vi "Combine Log of Mantissa and Exponent (SGL).vi"(5 "Exponent of 2":u8, 7 "10Log (Mantissa)":fxp<+/-,18,8>, 9 "Input Valid":bool=TRUE) -> (6 "Logarithm":fxp<+/-,34,12> format="%.26g", 10 "Output Valid":bool)   [LabVIEW 2012]
doc: "This VI implements the arithmetic of 10* log(M) + 10*log2* N\n\nOutput= 10Log(Matissa) + 3.01 *N\n\n<b> Resources Used: DSP48E</b>\n<b> Latency = 5 Ticks </b>"
uses:
  <vilib>/rvi/FXPMathLib/basic elements/DSP48E/simVIs/niFpgaDsp48eSimulationState.ctl
  <vilib>/rvi/FXPMathLib/basic elements/DSP48E/subVIs/niFpgaDsp48eType.ctl
  <vilib>/rvi/FXPMathLib/basic elements/DSP48E/subVIs/niFpgaDsp48eAlumodeOpmodeCarryinselState.ctl
  <vilib>/rvi/FXPMathLib/basic elements/DSP48E/subVIs/niFpgaDsp48eUseMultiplierState.ctl
  <vilib>/rvi/FXPMathLib/basic elements/DSP48E/subVIs/niFpgaDsp48eLogicUnitModeState.ctl
  <vilib>/rvi/FXPMathLib/basic elements/DSP48E/subVIs/niFpgaDsp48eSelectPatternState.ctl
  <vilib>/rvi/FXPMathLib/basic elements/DSP48E/subVIs/niFpgaDsp48eSelectMaskState.ctl
  <vilib>/rvi/FXPMathLib/basic elements/DSP48E/subVIs/niFpgaDsp48eAutoresetState.ctl
  <vilib>/rvi/FXPMathLib/basic elements/DSP48E/simVIs/niFpgaDsp48eResets.ctl
  <vilib>/rvi/FXPMathLib/basic elements/DSP48E/simVIs/niFpgaDsp48eEnables.ctl
  <vilib>/rvi/FXPMathLib/basic elements/DSP48E/simVIs/niFpgaDsp48eRegisters.ctl
  <vilib>/rvi/FXPMathLib/basic elements/DSP48E/simVIs/niFpgaDsp48eSimMultiplier.vi
  <vilib>/rvi/FXPMathLib/basic elements/DSP48E/simVIs/niFpgaDsp48eSimArithmetic.vi
  <vilib>/rvi/FXPMathLib/basic elements/DSP48E/simVIs/niFpgaDsp48eSimPatternDetect.vi
  <vilib>/rvi/FXPMathLib/basic elements/DSP48E/simVIs/niFpgaDsp48eSimP.vi
  <vilib>/rvi/FXPMathLib/basic elements/DSP48E/simVIs/niFpgaDsp48eSimUpdateState.vi
  <vilib>/rvi/FXPMathLib/basic elements/DSP48E/simVIs/niFpgaDsp48eCheckMode.vi
  <vilib>/rvi/FXPMathLib/basic elements/DSP48E/simVIs/niFpgaDsp48eReportInvalidMode.vi
  <vilib>/rvi/FXPMathLib/FxpInterpret/XNode/nifxpmath_Interpret.xnode
  <vilib>/rvi/FXPMathLib/basic elements/FxpDiscreteDelay/XNode/nifxpmath_DiscreteDelay.xnode
  <vilib>/rvi/FXPMathLib/basic elements/DSP48E/XNode/niFpgaDsp48e.xnode
panel:
  out "y":fxp<+/-,48,26>
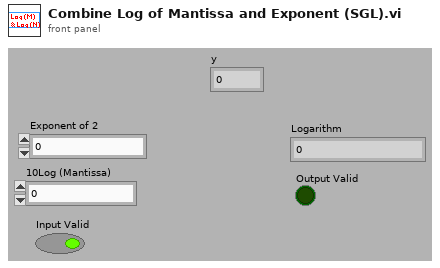
[diagram p1: front panel]
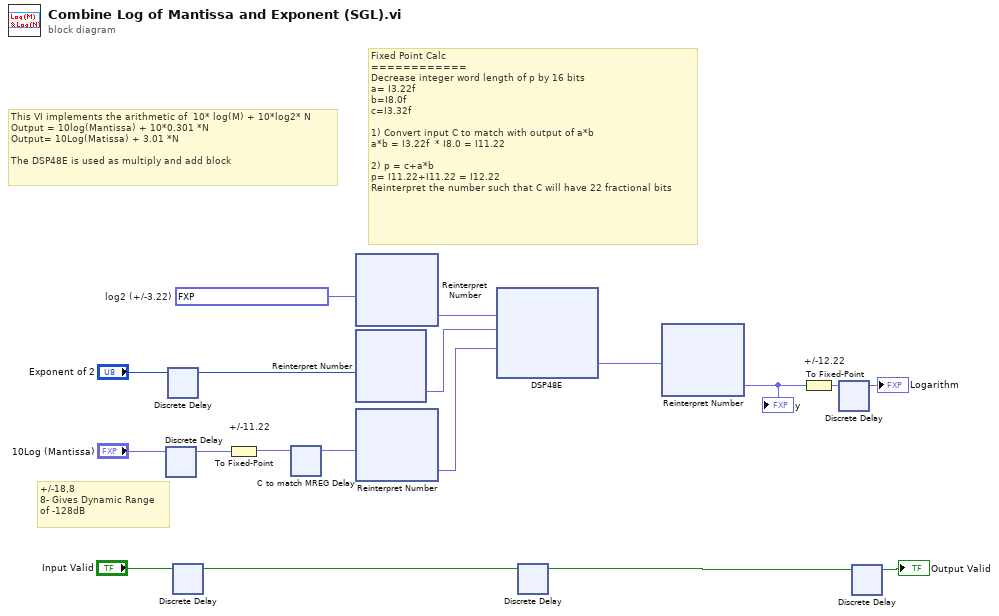
[diagram p0: block diagram]
diagram:
  w17 = fxp<+/-,25,3> 3.0102999210357666  # log2 (+/-3.22)
  # "This VI implements the arithmetic of  10* log(M) + 10*log2* N\nOutput = 10log(Mantissa) + 10*0.301 *N\nOutput= 10Log(Matissa) + 3.01 *N\n\nThe DSP48E is used as multiply and add block"
  # "+/-18,8\n8- Gives Dynamic Range\nof -128dB"
  # "Fixed Point Calc\n============\nDecrease integer word length of p by 16 bits\na= I3.22f\nb=I8.0f\nc=I3.32f\n\n1) Convert input C to match with output of a*b\na*b = I3.22f  * I8.0 = I11.22\n\n2) p = c+a*b\np= I11.22+I11.22 = I12.22\nReinterpret the number such that C will have 22 fractional bits"
  n1 = xnode ("Discrete Delay")("D"="10Log (Mantissa)") -> ("Q"=w2:fxp<+/-,18,8>)
  n2 = xnode ("Discrete Delay")("D"="Exponent of 2") -> ("Q"=w1:u8)
  n3 = xnode ("Discrete Delay")("D"="Input Valid") -> ("Q"=w3:bool)
  n4 = To Fixed-Point "+/-11.22"(number=w2) -> (fixed-point=w9:fxp<+/-,33,11>)  [unwired: 1 in]
  n5 = xnode "C to match MREG Delay"("D"=w9) -> ("Q"=w8:fxp<+/-,33,11>)
  n6 = xnode "Reinterpret Number"("x"=w17) -> ("y"=w18:fxp<+/-,25,25>)
  n7 = xnode "Reinterpret Number"("x"=w1) -> ("y"=w10:fxp<+/-,8,8>)
  n8 = xnode "Reinterpret Number"("x"=w8) -> ("y"=w12:fxp<+/-,33,33>)
  n9 = xnode ("DSP48E")("a"=w18, "b"=w10, "c"=w12) -> ("p"=w15:fxp<+/-,48,48>)
  n10 = xnode ("Discrete Delay")("D"=w3) -> ("Q"=w6:bool)
  n11 = xnode "Reinterpret Number"("x"=w15) -> ("y"=w14:fxp<+/-,48,26>)
  "y" <- w14
  n12 = To Fixed-Point "+/-12.22"(number=w14) -> (fixed-point=w13:fxp<+/-,34,12>)  [unwired: 1 in]
  n13 = xnode ("Discrete Delay")("D"=w13) -> ("Q"=→"Logarithm":fxp<+/-,34,12>)
  n14 = xnode ("Discrete Delay")("D"=w6) -> ("Q"=→"Output Valid":bool)
